vi "SVN_Revert.vi"(8 "error in (no error)":errorcluster, 10 "WorkingCopy":string) -> (0 "error out":errorcluster, 1 "command":string, 2 "standard output":string, 3 "standard error":string)   [LabVIEW 2017]
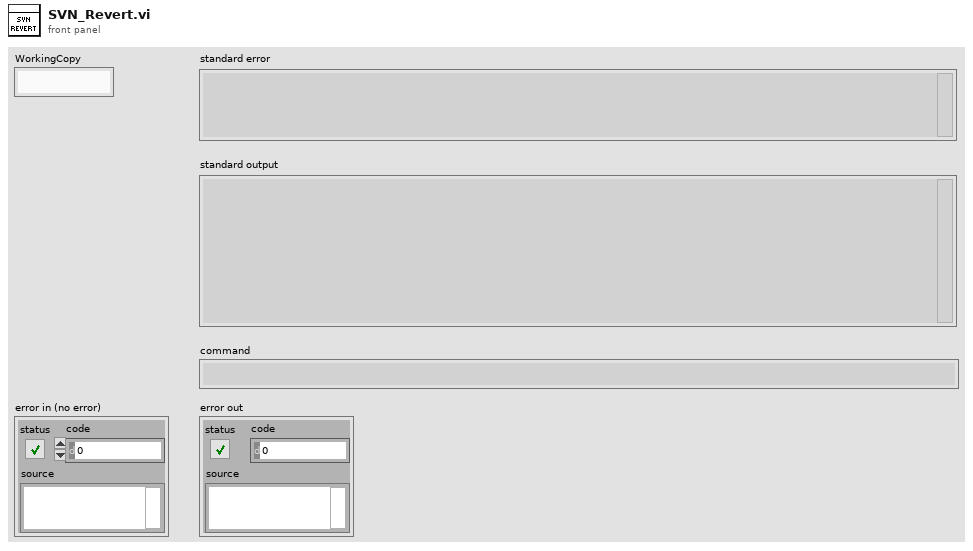
[diagram p1: front panel]
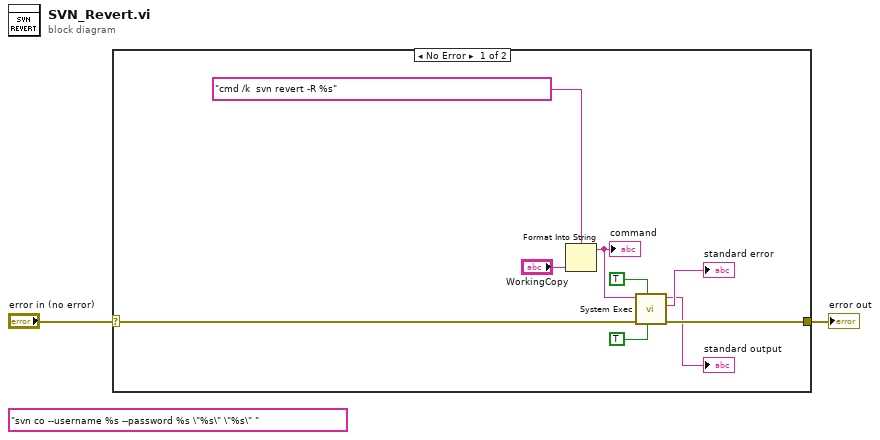
[diagram p0: block diagram]
diagram:
  (unwired) "svn co --username %s --password %s \"%s\" \"%s\" "
  n1 = case shown="No Error" "error in (no error)" {
    selector: "error in (no error)" -> [w10 w12]
    tunnel: [w11 w12] -> w2
    frame No Error {
      n2 = Format Into String(format string="cmd /k  svn revert -R %s", "WorkingCopy") -> (resulting string=w7:string)  [unwired: 2 in, 1 out]
      "command" <- w7
      n3 = call <vilib>:"System Exec.vi"("run minimized? (F)"=TRUE, "wait until completion? (T)"=TRUE, "error in (no error)"=w10, "command line"=w7) -> ("error out"=w11:errorcluster, "standard error"=→"standard error":string, "standard output"=→"standard output":string)  [unwired: 4 in, 1 out]
    }
    frame Error {
    }
  }
  "error out" <- w2
